vi "prepareToAck.vi"(8 "error in (no error)":errorcluster, 9 "cmdStatus":string(combo)="ack", 10 "cmd":string, 11 "tcpServerCmd in":refnum<class "TcpServerCmd.lvclass">) -> (0 "error out":errorcluster, 2 "JSON string":string, 3 "tcpServerCmd out":refnum<class "TcpServerCmd.lvclass">)   [LabVIEW 2018, in "TcpServerCmd.lvclass"]
doc: "Prepare the command received to do the acknowledgement to TCP Client."
uses:
  TcpServerCmd.lvclass
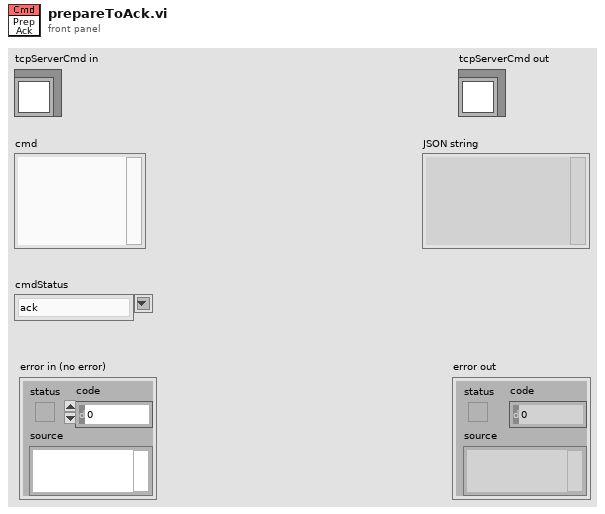
[diagram p1: front panel]
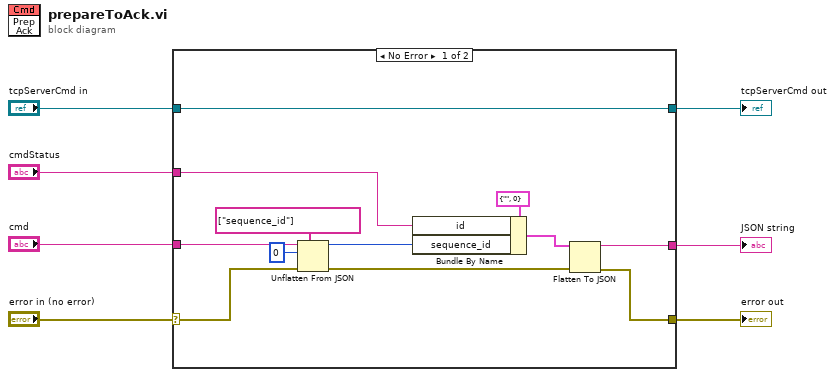
[diagram p0: block diagram]
diagram:
  n1 = case shown="No Error" "error in (no error)" {
    selector: "error in (no error)" -> [w12 w21]
    tunnel: [w10 w21] -> w6
    tunnel: [w19 w20] -> w4
    tunnel: "tcpServerCmd in" -> [w19 w20]
    tunnel: "cmd" -> [w17 _]
    tunnel: [w13 _] -> w2
    tunnel: "cmdStatus" -> [w8 _]
    frame No Error {
      n2 = Unflatten From JSON(path=string[] ["sequence_id"], JSON string=w17, type and defaults=0, error in (no error)=w12) -> (value=w9:i32, error out=w11:errorcluster)  [unwired: 3 in]
      n3 = Bundle By Name(cluster=cluster{"id":string, "sequence_id":i32} {"id"="", "sequence_id"=0}, "id"=w8, "sequence_id"=w9) -> (w14:cluster{"id":string, "sequence_id":i32})
      n4 = Flatten To JSON(anything=w14, error in (no error)=w11) -> (JSON string=w13:string, 11:w10:errorcluster)  [unwired: 1 in]
    }
    frame Error {
    }
  }
  "error out" <- w6
  "tcpServerCmd out" <- w4
  "JSON string" <- w2
